vi "Get Homed Status.vi"(8 "error in (no error)":errorcluster, 10 "Axis":string, 11 "SIM Motion Controller in":refnum<class "Fine SIM Motion Controller.lvclass">) -> (0 "error out":errorcluster, 2 "Homed?":bool, 3 "SIM Motion Controller out":refnum<class "Fine SIM Motion Controller.lvclass">)   [LabVIEW 2022 SP3, in "Fine SIM Motion Controller.lvclass"]
uses:
  Fine SIM Motion Controller.lvclass
  Fine SIM Motion Controller.lvclass/Fine SIM Motion Controller.ctl
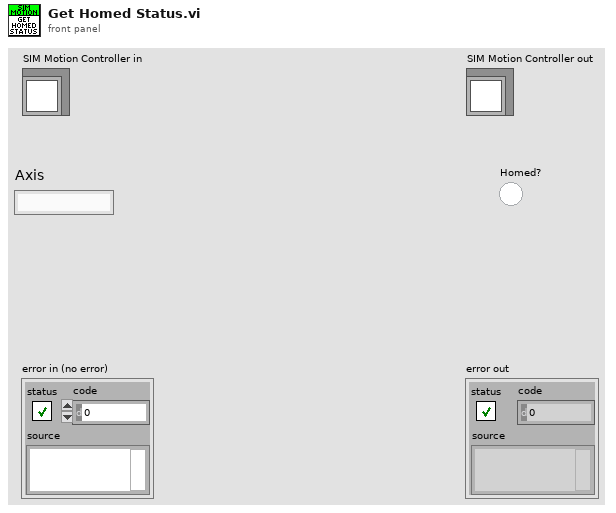
[diagram p1: front panel]
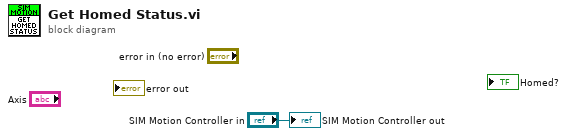
[diagram p0: block diagram]
diagram:
  "SIM Motion Controller out" <- "SIM Motion Controller in"
